vi "解析表格mark.vi"(0 "点位信息表":string[][](table)=[["PCB1-拍照点1(Mark1)", "-73.376", "-164.238", "0.000", "-103.848", "565.620", "384.924", "377.049", "0.000", "0.000", "0.000", "0", "8", "94", "1"], ["PCB1-拍照点2(Mark2)", "-260.376", "-49.239", "0.000", "-290.450", "681.264", "384.924", "377.049", "0.000", "0.000", "0.000", "-180", "8", "94", "1"], ["拍照点3", "-73.376", "-49.239", "0.000", "-103.451", "680.618", "384.924", "377.049", "0.000", "0.000", "0.000", "0", "8", "94", "1"], ["拍照点4", "-260.376", "-164.238", "0.000", "-290.847", "566.266", "384.924", "377.049", "0.000", "0.000", "0.000", "-180", "8", "94", "1"], ["拍照点5", "-260.376", "-104.239", "0.000", "-290.640", "626.265", "384.924", "377.049", "0.000", "0.000", "0.000", "-180", "8", "94", "1"], ["拍照点6", "-240.876", "-23.738", "0.000", "-270.862", "706.698", "384.924", "377.049", "0.000", "0.000", "0.000", "90", "8", "94", "1"], ["拍照点7", "-190.876", "-23.738", "0.000", "-220.862", "706.525", "384.924", "377.049", "0.000", "0.000", "0.000", "90", "8", "94", "0"], ["拍照点8", "-142.876", "-23.738", "0.000", "-172.862", "706.359", "384.924", "377.049", "0.000", "0.000", "0.000", "90", "8", "94", "0"], ["拍照点9", "-92.876", "-23.738", "0.000", "-122.863", "706.187", "384.924", "377.049", "0.000", "0.000", "0.000", "90", "8", "94", "0"], ["拍照点10", "-73.376", "-104.239", "0.000", "-103.641", "625.619", "384.924", "377.049", "0.000", "0.000", "0.000", "0", "8", "94", "0"], ["拍照点11", "-112.876", "-169.238", "0.000", "-143.365", "560.756", "384.924", "377.049", "0.000", "0.000", "0.000", "-90", "8", "94", "0"], ["拍照点12", "-220.876", "-169.238", "0.000", "-251.364", "561.130", "384.924", "377.049", "0.000", "0.000", "0.000", "0", "8", "94", "0"], ["PCB2-拍照点1(Mark3)", "-73.376", "-164.238", "0.000", "151.457", "565.201", "384.924", "377.049", "0.000", "0.000", "-3.000", "0", "8", "94", "1"], ["PCB2-拍照点2(Mark4)", "-260.376", "-49.239", "0.000", "-35.509", "680.255", "384.924", "377.049", "0.000", "0.000", "-3.000", "-180", "8", "94", "1"], ["拍照点3", "-73.376", "-49.239", "0.000", "151.491", "680.200", "384.924", "377.049", "0.000", "0.000", "-3.000", "0", "8", "94", "1"], ["拍照点4", "-260.376", "-164.238", "0.000", "-35.543", "565.256", "384.924", "377.049", "0.000", "0.000", "-3.000", "-180", "8", "94", "1"], ["拍照点5", "-260.376", "-104.239", "0.000", "-35.525", "625.255", "384.924", "377.049", "0.000", "0.000", "-3.000", "-180", "8", "94", "1"], ["拍照点6", "-240.876", "-23.738", "0.000", "-16.001", "705.751", "384.924", "377.049", "0.000", "0.000", "-3.000", "90", "8", "94", "1"], ["拍照点7", "-190.876", "-23.738", "0.000", "33.999", "705.736", "384.924", "377.049", "0.000", "0.000", "0.000", "90", "8", "94", "0"], ["拍照点8", "-142.876", "-23.738", "0.000", "81.999", "705.722", "384.924", "377.049", "0.000", "0.000", "0.000", "90", "8", "94", "0"], ["拍照点9", "-92.876", "-23.738", "0.000", "131.999", "705.707", "384.924", "377.049", "0.000", "0.000", "0.000", "90", "8", "94", "0"], ["拍照点10", "-73.376", "-104.239", "0.000", "151.475", "625.200", "384.924", "377.049", "0.000", "0.000", "0.000", "0", "8", "94", "0"], ["拍照点11", "-112.876", "-169.238", "0.000", "111.956", "560.213", "384.924", "377.049", "0.000", "0.000", "0.000", "-90", "8", "94", "0"], ["拍照点12", "-220.876", "-169.238", "0.000", "3.956", "560.245", "384.924", "377.049", "0.000", "0.000", "0.000", "0", "8", "94", "0"]]) -> (4 "基本信息":T1, 6 "布线前甩线":string[][](table), 8 "布线点位":string[][](table), 10 "布线后甩线":string[][](table), 15 "进出线编码":cluster{"进线编码":i32, "出线编码":i32}[](array[cluster]))   [LabVIEW 2014]
uses:
  Global.vi
panel:
  out "甩线后":dbl[](array[numeric])
  out "布线":dbl[](array[numeric])
  out "甩线前":dbl[](array[numeric])
  out "线号ok":bool
  out "数据正常":bool
  in  "基本信息":T1
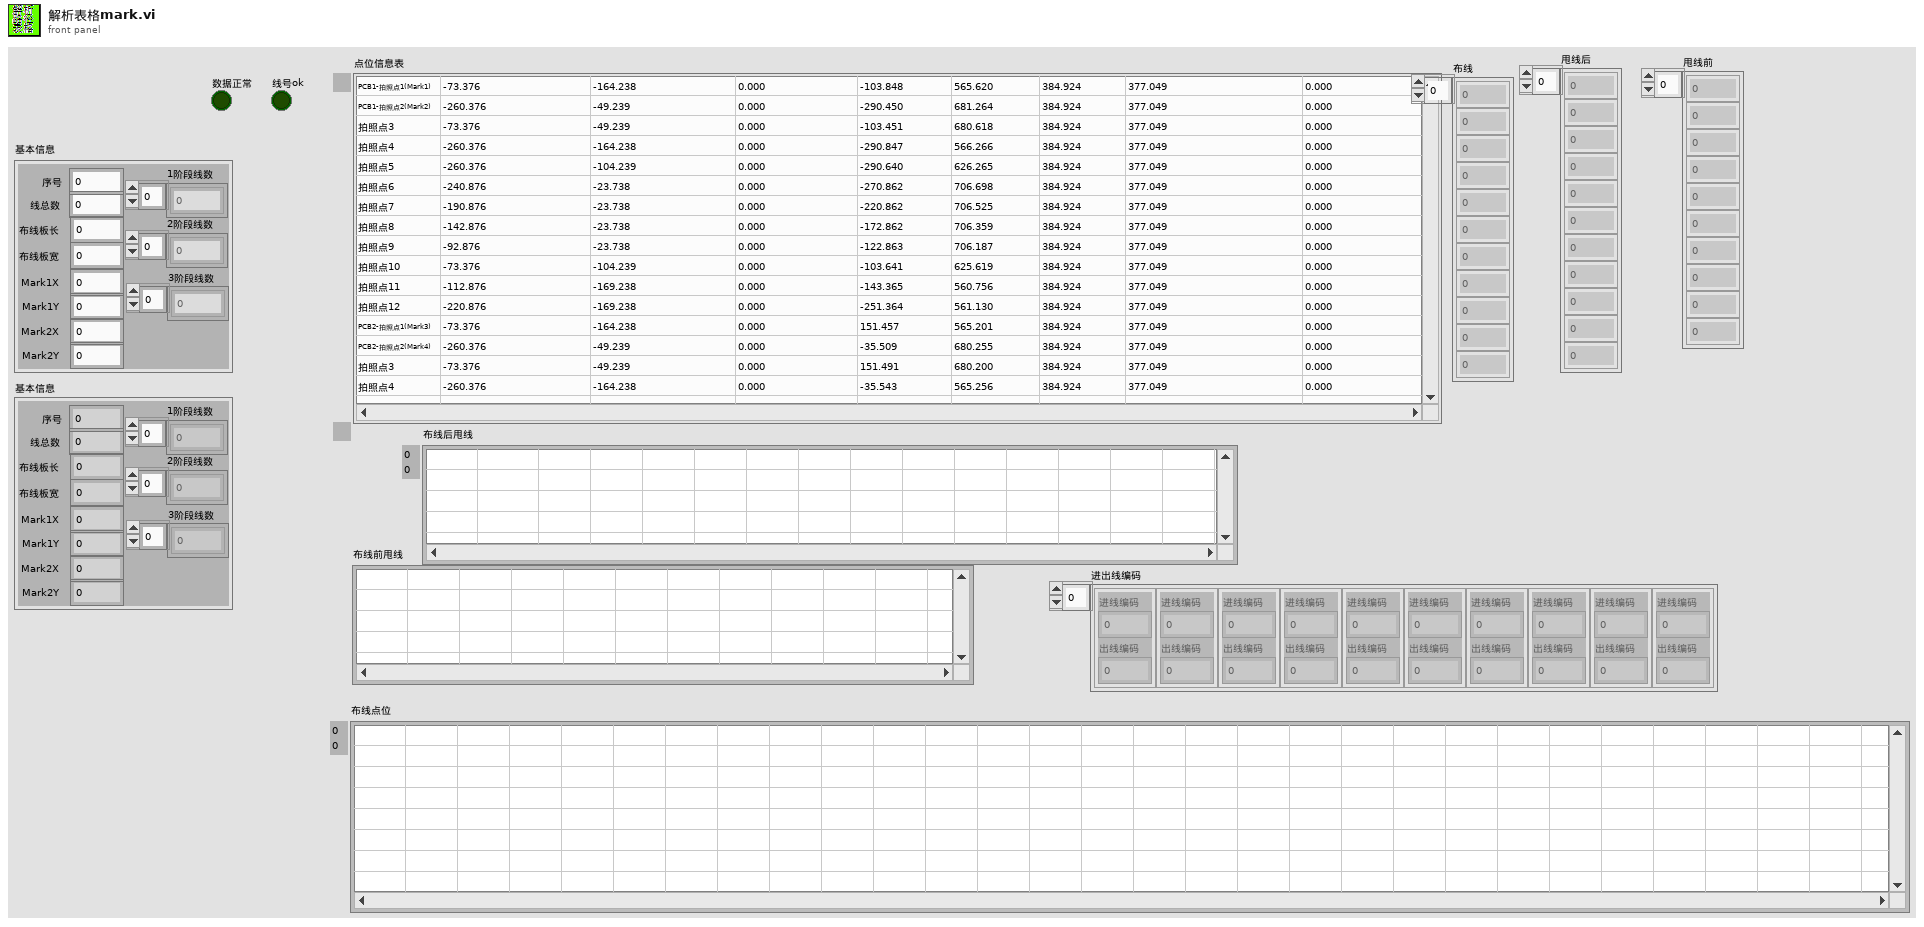
[diagram p1: front panel]
types:
  T1 = typedef "基本信息.ctl" = cluster{"序号":dbl, "线总数":dbl, "布线板长":dbl, "布线板宽":dbl, "Mark1X":dbl, "Mark1Y":dbl, "Mark2X":dbl, "Mark2Y":dbl, "1阶段线数":dbl[], "2阶段线数":dbl[], "3阶段线数":dbl[]}
  T2 = typedef "XYPos.ctl" = cluster{"X":dbl, "Y":dbl}
  T3 = typedef "mark规格.ctl" = cluster{"X下限":dbl, "X上限":dbl, "Y下限":dbl, "Y 上限":dbl, "angle下限":dbl, "angle上限":dbl}
  T4 = cluster{"甩线补偿值":cluster{"下边":dbl, "距离上边":dbl, "左边":dbl, "右边":dbl}, "补偿甩线坐标偏移":T2, "mark点模组补偿":T2, "出线补偿值":dbl, "mark规格":T3}
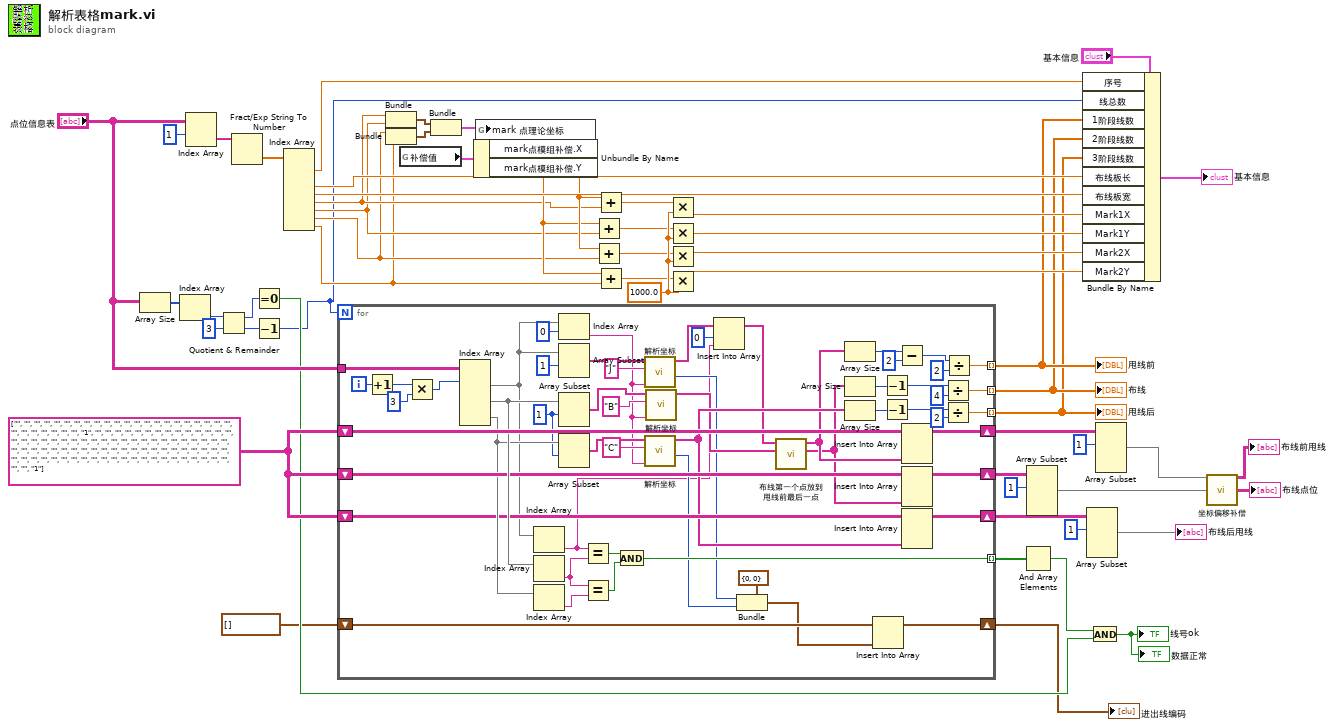
[diagram p0: block diagram]
diagram:
  w18 = 1000.0 ("y")
  w48 = string[][] [["", "", "", "", "", "", "", "", "", "", "", "", "", "", "", "", "", "", "", "", "", "", "", "", "", "", "", "", "", "1", "", "", "", "", "", "", "", "", "", "", "", "", "", "", "", "", "", "", "", "", "", "", "", "", "", "", "", "", "", "", "", "", "", "", "", "", "", "", "", "", "", "", "", "", "", "", "", "", "", "", "", "", "", "", "", "", "", "", "", "", "", "", "", "", "", "", "", "", "", "", "", "", "", "", "", "", "", "", "", "", "", "", "1"]]
  n1 = Array Size(array="点位信息表") -> (size(s)=w52:i32[])
  n2 = Index Array(array=w52) -> (element=w51:i32)  [unwired: 1 in]
  n3 = Index Array(array="点位信息表", index (row)=1 ("索引 (行)")) -> (element=w54:string[])  [unwired: 1 in]
  n4 = Quotient & Remainder(x=w51, y=3) -> (x-y*floor(x/y)=w49:i32, floor(x/y)=w46:i32)
  n5 = Fract/Exp String To Number(string=w54) -> (number=w45:dbl[])  [unwired: 3 in, 1 out]
  n6 = Equal To 0?(x=w49) -> (x = 0?=w36:bool)
  n7 = Decrement(x=w46) -> (x-1=w2:i32)
  n8 = Index Array(array=w45) -> (element #1=w31:dbl, element #3=w44:dbl, element #4=w43:dbl, element #5=w11:dbl, element #6=w10:dbl, element #7=w6:dbl, element #8=w5:dbl)  [unwired: 8 in, 1 out]
  n9 = for {
    N: w2 -> [_]
    tunnel: "点位信息表" -> [w111]
    tunnel: [w102] -> w38 mode=indexing
    shift-right: [w98] -> w30
    shift-left: w48 -> [w101]
    shift-right: [w89] -> w25
    shift-left: w48 -> [w94]
    shift-right: [w88] -> w26
    shift-left: w48 -> [w87]
    tunnel: [w85] -> w34 mode=indexing
    tunnel: [w81] -> w33 mode=indexing
    tunnel: [w80] -> w32 mode=indexing
    shift-right: [w67] -> w19
    shift-left: cluster{"进线编码":i32, "出线编码":i32}[] [] -> [w69]
    i -> [w110]
    w73 = 1 ("索引")
    n10 = Increment(x=w110) -> (x+1=w107:i32)
    n11 = Multiply(x=w107, y=3) -> (x*y=w108:i32)
    n12 = Index Array(array=w111, index (row) #1=w108) -> (element #1=w76:string[], element #2=w97:string[], element #3=w92:string[])  [unwired: 5 in]
    n13 = Index Array(array=w76) -> (element=w60:string)  [unwired: 1 in]
    n14 = Index Array(array=w97) -> (element=w106:string)  [unwired: 1 in]
    n15 = Index Array(array=w92) -> (element=w105:string)  [unwired: 1 in]
    n16 = Index Array(array=w76, index=0 ("索引")) -> (element=w74:string)
    n17 = Array Subset(array=w76, index=1 ("索引")) -> (w100:string[])  [unwired: 1 in]
    n18 = Array Subset(array=w97, index=w73) -> (w95:string[])  [unwired: 1 in]
    n19 = Array Subset(array=w92, index=w73) -> (w91:string[])  [unwired: 1 in]
    n20 = Equal?(x=w60, y=w106) -> (x = y?=w104:bool)
    n21 = Equal?(x=w106, y=w105) -> (x = y?=w103:bool)
    n22 = And(x=w104, y=w103) -> (x .and. y?=w102:bool)
    n23 = call "解析坐标.vi"("线号"=w74, "匹配字符"="J", "解析数组"=w100) -> ("编码数值"=w72:i32, "坐标xy顺序"=w62:string[])  [unwired: 6 in, 1 out]
    n24 = call "解析坐标.vi"("线号"=w74, "匹配字符"="C", "解析数组"=w91) -> ("编码数值"=w71:i32, "坐标xy顺序"=w83:string[])  [unwired: 6 in, 1 out]
    n25 = call "解析坐标.vi"("线号"=w74, "匹配字符"="B", "解析数组"=w95) -> ("坐标xy顺序"=w79:string[])  [unwired: 6 in, 2 out]
    n26 = Insert Into Array(array=w62, index=0 ("索引"), new element=w60) -> (w61:string[])
    n27 = Bundle(cluster=cluster{"进线编码":i32, "出线编码":i32} {"进线编码"=0, "出线编码"=0}, "进线编码"=w72, "出线编码"=w71) -> (w68:cluster{"进线编码":i32, "出线编码":i32})
    n28 = call "布线第一个点放到甩线前最后一点.vi"("布线点"=w79, "甩线前"=w61) -> ("布线点 2"=w77:string[], "甩线前 2"=w78:string[])  [unwired: 8 in]
    n29 = Array Size(array=w78) -> (size(s)=w66:i32)
    n30 = Array Size(array=w77) -> (size(s)=w59:i32)
    n31 = Array Size(array=w83) -> (size(s)=w57:i32)
    n32 = Insert Into Array(array=w69, new element=w68) -> (w67:cluster{"进线编码":i32, "出线编码":i32}[])  [unwired: 1 in]
    n33 = Decrement(x=w59) -> (x-1=w58:i32)
    n34 = Decrement(x=w57) -> (x-1=w56:i32)
    n35 = Subtract(x=w66, y=2) -> (x-y=w65:i32)
    n36 = Insert Into Array(array=w101, new element=w78) -> (w98:string[][])  [unwired: 2 in]
    n37 = Insert Into Array(array=w94, new element=w77) -> (w89:string[][])  [unwired: 2 in]
    n38 = Insert Into Array(array=w87, new element=w83) -> (w88:string[][])  [unwired: 2 in]
    n39 = Divide(x=w58, y=4) -> (x/y=w81:dbl)
    n40 = Divide(x=w56, y=2) -> (x/y=w80:dbl)
    n41 = Divide(x=w65, y=2) -> (x/y=w85:dbl)
  }
  "甩线前" <- w34
  "布线" <- w33
  "甩线后" <- w32
  "进出线编码" <- w19
  n42 = Bundle(w11, w10) -> (w8:cluster{dbl, dbl})  [unwired: 1 in]
  n43 = Bundle(w6, w5) -> (w7:cluster{dbl, dbl})  [unwired: 1 in]
  n44 = global read "Global.vi" "补偿值"() -> (w1:T4)
  n45 = Bundle(w8, w7) -> (w9:cluster{cluster{dbl, dbl}, cluster{dbl, dbl}})  [unwired: 1 in]
  n46 = Unbundle By Name(w1) -> ("mark点模组补偿.X"=w14:dbl, "mark点模组补偿.Y"=w12:dbl)
  n47 = global write "Global.vi" "mark 点理论坐标"(w9) -> ()
  n48 = Add(x=w12, y=w10) -> (x+y=w16:dbl)
  n49 = Add(x=w14, y=w6) -> (x+y=w15:dbl)
  n50 = Add(x=w14, y=w11) -> (x+y=w17:dbl)
  n51 = Add(x=w12, y=w5) -> (x+y=w13:dbl)
  n52 = Multiply(x=w17, y=w18) -> (x*y=w42:dbl)
  n53 = Multiply(x=w16, y=w18) -> (x*y=w41:dbl)
  n54 = Multiply(x=w15, y=w18) -> (x*y=w40:dbl)
  n55 = Multiply(x=w13, y=w18) -> (x*y=w39:dbl)
  n56 = And Array Elements(Boolean array=w38) -> (logical AND=w37:bool)
  n57 = Array Subset(array=w25, index (row)=1 ("索引")) -> (w22:string[][])  [unwired: 3 in]
  n58 = Bundle By Name(cluster="基本信息", "序号"=w31, "线总数"=w2, "1阶段线数"=w34, "2阶段线数"=w33, "3阶段线数"=w32, "布线板长"=w44, "布线板宽"=w43, "Mark1X"=w42, "Mark1Y"=w41, "Mark2X"=w40, "Mark2Y"=w39) -> (→"基本信息":T1)
  n59 = Array Subset(array=w26, index (row)=1 ("索引")) -> (→"布线后甩线":string[][])  [unwired: 3 in]
  n60 = And(x=w37, y=w36) -> (x .and. y?=→"数据正常" →"线号ok":bool)
  n61 = Array Subset(array=w30, index (row)=1 ("索引")) -> (w4:string[][])  [unwired: 3 in]
  n62 = call "坐标偏移补偿.vi"("布线前甩线"=w4, "布线点位"=w22) -> ("布线前甩线矫正后"=→"布线前甩线":string[][], "布线点矫正后"=→"布线点位":string[][])  [unwired: 11 in, 1 out]
